vi "G#Object_RunVI.vi"(0 "vi reference":refnum<vi>, 1 "control names":string[](array[string]), 3 "control values":variant[](array[variant]), 5 "error in (no error)":errorcluster) -> (18 "error out from VI":errorcluster, 19 "error out":errorcluster)   [LabVIEW 2020, in "G#Object.lvclass"]
doc: "Runs the VI specified by the vi reference."
uses:
  <vilib>/addons/_AddQ/G#Object/G#Object.lvclass
  <vilib>/addons/_AddQ/G#Object/utils/G#Object_EventType.ctl
  <vilib>/addons/_AddQ/G#Object/utils/G#Object_ObjectInfoType.ctl
  <vilib>/addons/_AddQ/G#Object/utils/G#Object_CreateMethod.ctl
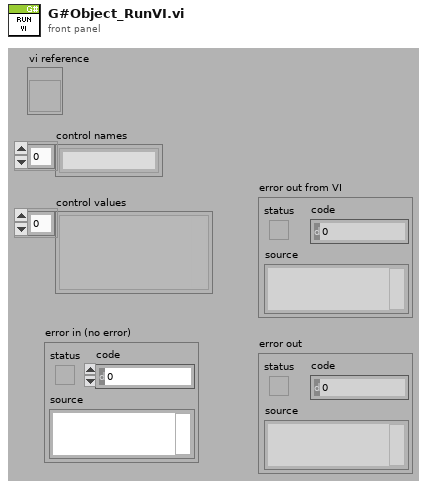
[diagram p1: front panel]
types:
  T1 = typedef "G#Object.lvclass/G#Object_ObjectInfoType.ctl" = cluster{"ObjectName":string, "ObjectID":u32, "Users":i32, "Counter":bool, "AttributeRefs":u32[], "FullClassName":string, "ClassName":string, "CreateMethod":T2, "GenericDestructorExists":bool, "Owner":string}
  T2 = typedef "G#Object.lvclass/G#Object_CreateMethod.ctl" = enum16{"Create", "Create or look up existing", "Look up existing"}
  T3 = typedef "G#Object.lvclass/G#Object_EventType.ctl" = enum16{"Created new", "Looked up existing", "Deleted", "Forced delete", "Not deleted", "Garbage collected", "Cleared", "User", "Error", "External create object", "External create class attributes", "Created class attributes", "Run constructor", "Run constructor done", "Run open method", "Run open method done"}
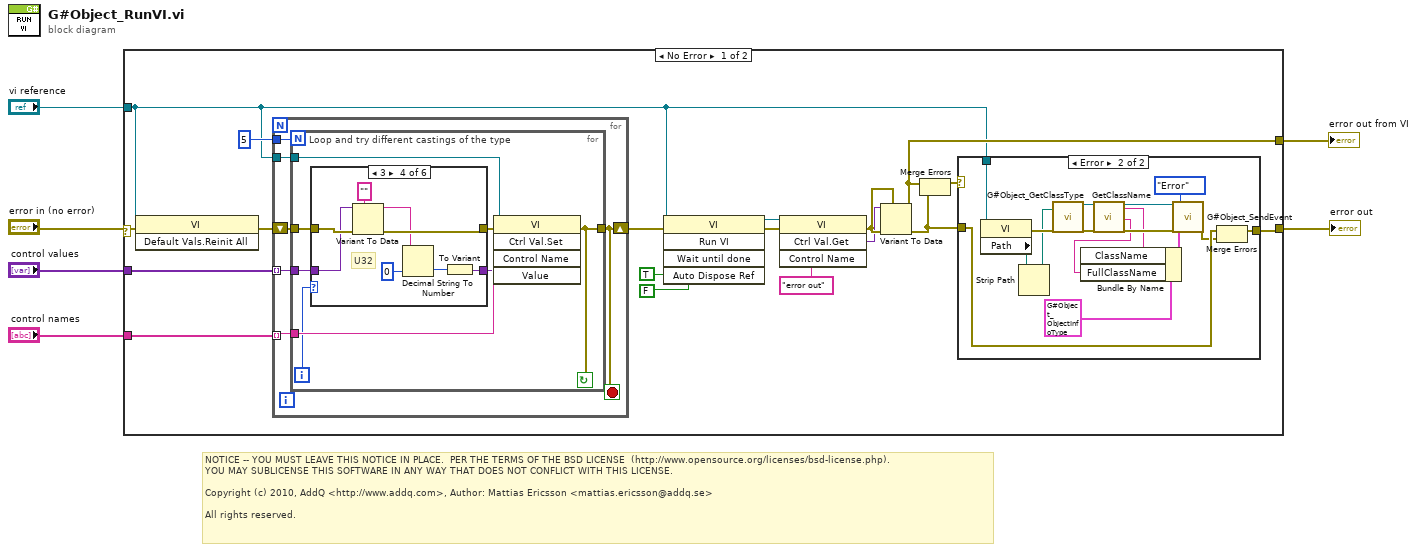
[diagram p0: block diagram]
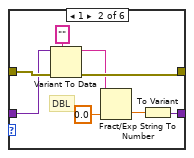
[diagram p4: hidden frame]
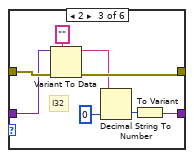
[diagram p5: hidden frame]
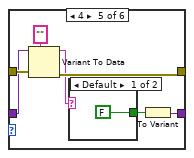
[diagram p6: hidden frame]
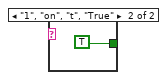
[diagram p7: hidden frame]
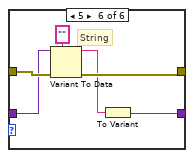
[diagram p8: hidden frame]
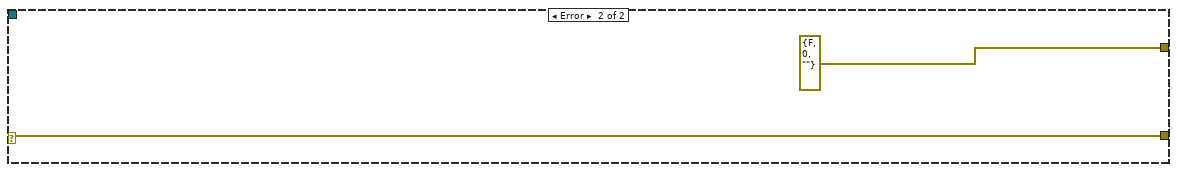
[diagram p9: hidden frame]
diagram:
  # "NOTICE -- YOU MUST LEAVE THIS NOTICE IN PLACE.  PER THE TERMS OF THE BSD LICENSE  (http://www.opensource.org/licenses/bsd-license.php).\nYOU MAY SUBLICENSE THIS SOFTWARE IN ANY WAY THAT DOES NOT CONFLICT WITH THIS LICENSE.\n\nCopyright (c) 2010, AddQ <http://www.addq.com>, Author: Mattias Ericsson <mattias.ericsson@addq.se>\n\nAll rights reserved."
  n1 = case shown="No Error" "error in (no error)" {
    selector: "error in (no error)" -> [w15 w98]
    tunnel: "vi reference" -> [w11 _]
    tunnel: "control values" -> [w19 _]
    tunnel: "control names" -> [w18 _]
    tunnel: [w13 errorcluster {"status"=FALSE, "code"=0, "source"=""} ("error out")] -> w3
    tunnel: [w10 w98] -> w2
    frame No Error {
      n2 = invoke class="VI" method="Default Vals.Reinit All"(reference=w11, error in=w15) -> (error out=w24:errorcluster)  [unwired: 1 in, 2 out]
      n3 = for {
        shift-right: [w42] -> w8
        shift-left: w24 -> [w47]
        tunnel: w11 -> [w46]
        tunnel: w18 -> [w45] mode=indexing
        tunnel: w19 -> [w44] mode=indexing
        tunnel: 5 -> [w43]
        stop <- w42 stop-if-true
        n4 = for {
          N: w43 -> [_]
          tunnel: w47 -> [w50]
          tunnel: w46 -> [w55]
          tunnel: w45 -> [w54]
          tunnel: w44 -> [w52]
          tunnel: [w48] -> w42
          i -> [w53]
          stop <- w48 continue-if-true
          # "Loop and try different castings of the type"
          n5 = case shown="3" w53 {
            tunnel: [w57 w62 w70 w78 w85 w93] -> w51
            tunnel: w52 -> [w57 w64 w72 w80 w87 w95]
            tunnel: w50 -> [w56 w65 w73 w81 w88 w96]
            tunnel: [w56 w63 w71 w79 w86 w94] -> w49
            frame 0, Default {
            }
            frame 1 {
              # "DBL"
              n6 = Variant To Data(error in=w65, type="" ("y"), Variant=w64) -> (data=w60:string, error out=w63:errorcluster)
              n7 = Fract/Exp String To Number(string=w60, default (0 dbl)=0.0 ("default (0 DBL)")) -> (number=w59:dbl)  [unwired: 2 in, 1 out]
              n8 = To Variant(anything=w59) -> (Variant=w62:variant)
            }
            frame 2 {
              # "I32"
              n9 = Variant To Data(error in=w73, type="" ("y"), Variant=w72) -> (data=w68:string, error out=w71:errorcluster)
              n10 = Decimal String To Number(string=w68, default (0L)=0 ("default (0 DBL)")) -> (number=w67:i32)  [unwired: 1 in, 1 out]
              n11 = To Variant(anything=w67) -> (Variant=w70:variant)
            }
            frame 3 {
              # "U32"
              n12 = Variant To Data(error in=w81, type="" ("y"), Variant=w80) -> (data=w76:string, error out=w79:errorcluster)
              n13 = Decimal String To Number(string=w76, default (0L)=u32 0 ("default (0 DBL)")) -> (number=w75:u32)  [unwired: 1 in, 1 out]
              n14 = To Variant(anything=w75) -> (Variant=w78:variant)
            }
            frame 4 {
              n15 = Variant To Data(error in=w88, type="" ("y"), Variant=w87) -> (data=w83:string, error out=w86:errorcluster)
              n16 = case shown="Default" w83 {
                tunnel: [FALSE TRUE] -> w82
                frame Default {
                }
                frame "1", "on", "t", "True" {
                }
              }
              n17 = To Variant(anything=w82) -> (Variant=w85:variant)
            }
            frame 5 {
              # "String"
              n18 = Variant To Data(error in=w96, type="", Variant=w95) -> (data=w91:string, error out=w94:errorcluster)
              n19 = To Variant(anything=w91) -> (Variant=w93:variant)
            }
          }
          n20 = invoke class="VI" method="Ctrl Val.Set"(reference=w55, error in=w49, "Control Name"=w54, "Value"=w51) -> (error out=w48:errorcluster)  [unwired: 1 in, 4 out]
        }
      }
      n21 = invoke class="VI" method="Run VI"(reference=w11, error in=w8, "Wait until done"=TRUE ("Wait Until Done"), "Auto Dispose Ref"=FALSE ("Auto Dispose Reference")) -> (reference out=w20:refnum<vi>, error out=w7:errorcluster)  [unwired: 1 in, 3 out]
      n22 = invoke class="VI" method="Ctrl Val.Get"(reference=w20, error in=w7, "Control Name"="error out") -> (error out=w23:errorcluster, "Get Control Value Variant"=w22:variant)  [unwired: 1 in, 2 out]
      n23 = Variant To Data(error in=w23, type=w23, Variant=w22) -> (data=w13:errorcluster, error out=w9:errorcluster)
      n24 = Merge Errors(w13, w9) -> (w12:errorcluster)
      n25 = case shown="Error" w12 {
        tunnel: w11 -> [_ w39]
        tunnel: [w25 w29] -> w10
        tunnel: w9 -> [w25 w28]
        frame No Error {
        }
        frame Error {
          n26 = property class="VI"(reference=w39) -> (error out=w40:errorcluster, "Path"=w38:path)  [unwired: 1 in, 1 out]
          n27 = Strip Path(path=w38) -> (stripped path=w37:path)  [unwired: 1 out]
          n28 = call <vilib>:"G#Object_GetClassType.vi"("class path"=w37, "error in (no error)"=w40) -> ("reference out"=w36:refnum<class "G#Object.lvclass">, "error out"=w35:errorcluster)  [unwired: 16 in]
          n29 = call-dynamic "GetClassName.vi"("reference in"=w36, "error in (no error)"=w35) -> ("reference out"=w34:refnum<class "G#Object.lvclass">, "class name"=w30:string, "full class name"=w26:string, "error out"=w31:errorcluster)  [unwired: 13 in, 1 out]
          n30 = Bundle By Name(cluster=T1 {"ObjectName"="", "ObjectID"=0, "Users"=0, "Counter"=FALSE, "AttributeRefs"=[], "FullClassName"="", "ClassName"="", "CreateMethod"=enum."Create", "GenericDestructorExists"=FALSE, "Owner"=""} ("object info extended"), "ClassName"=w30, "FullClassName"=w26) -> (w32:T1)
          n31 = call <vilib>:"G#Object_SendEvent.vi"("reference in"=w34, "object info extended"=w32, "error in (no error)"=w31, "G# event type"=G#Object_EventType."Error" ("G#Event")) -> ("error out"=w27:errorcluster)  [unwired: 15 in]
          n32 = Merge Errors(w28, w27) -> (w29:errorcluster)
        }
      }
    }
    frame Error {
    }
  }
  "error out" <- w2
  "error out from VI" <- w3
